vi "PositionInterpolator.vi"() -> ()   [LabVIEW 2013]
panel:
  out "Positions":dbl[](array[numeric])
  in  "timestamp":dbl format="%#_13g"
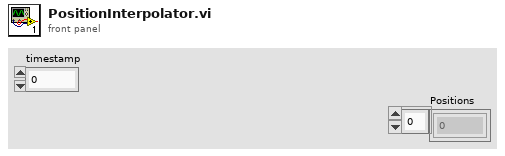
[diagram p1: front panel]
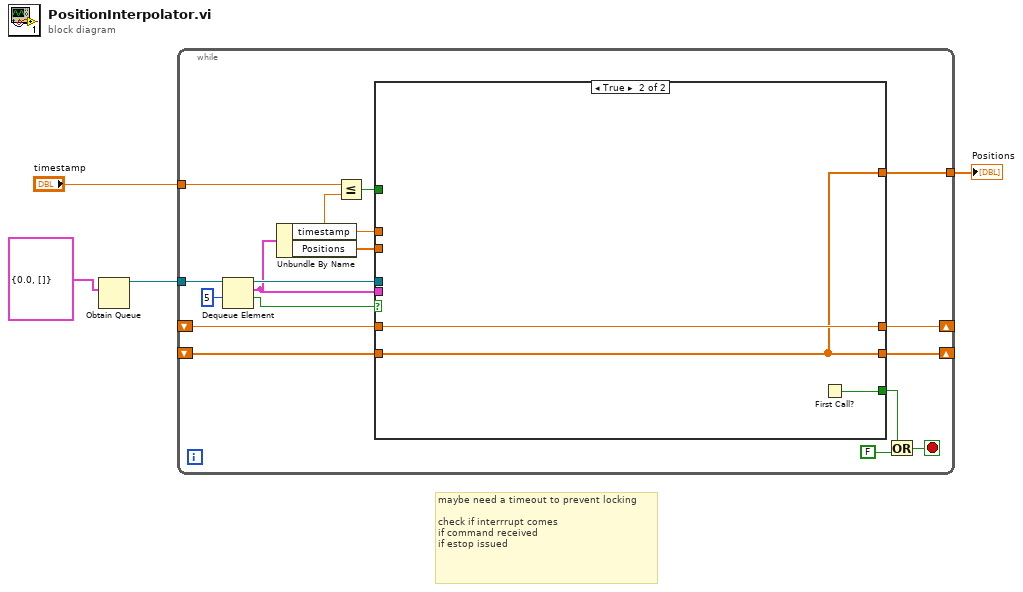
[diagram p0: block diagram]
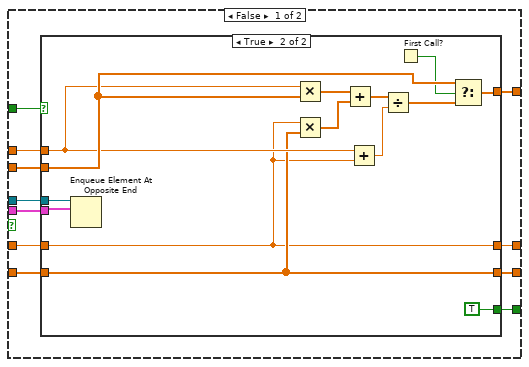
[diagram p2: hidden frame]
diagram:
  # "maybe need a timeout to prevent locking\n\ncheck if interrrupt comes\nif command received\nif estop issued"
  n1 = Obtain Queue(element data type=cluster{"timestamp":dbl, "Positions":dbl[]} {"timestamp"=0.0, "Positions"=[]}) -> (queue out=w3:refnum<queue>)  [unwired: 4 in, 2 out]
  n2 = while {
    tunnel: w3 -> [w21]
    tunnel: "timestamp" -> [w18]
    tunnel: [w14] -> w1
    shift-right: [w12] -> _
    shift-left: _ -> [w9]
    shift-right: [w11] -> _
    shift-left: _ -> [w10]
    stop <- w8 stop-if-true
    n3 = Dequeue Element(queue=w21, timeout in ms (-1)=5) -> (queue out=w20:refnum<queue>, element=w6:cluster{"timestamp":dbl, "Positions":dbl[]}, timed out?=w5:bool)  [unwired: 1 in, 1 out]
    n4 = Unbundle By Name(w6) -> ("timestamp"=w15:dbl, "Positions"=w16:dbl[])
    n5 = Less Or Equal?(x=w18, y=w15) -> (x <= y?=w17:bool)
    n6 = case shown="True" w5 {
      tunnel: w20 -> [w32 _]
      tunnel: w17 -> [w31 _]
      tunnel: w16 -> [w30 _]
      tunnel: w15 -> [w29 _]
      tunnel: [w28 w50] -> w14
      tunnel: [w27 w49] -> w13
      tunnel: [w26 w50] -> w12
      tunnel: [w25 w51] -> w11
      tunnel: w10 -> [w24 w51]
      tunnel: w9 -> [w23 w50]
      tunnel: w6 -> [w22 _]
      frame False {
        n7 = case shown="True" w31 {
          tunnel: w32 -> [_ w36]
          tunnel: w30 -> [w34 w41]
          tunnel: w29 -> [w33 w40]
          tunnel: [_ w43] -> w28
          tunnel: [_ TRUE] -> w27
          tunnel: [w34 w38] -> w26
          tunnel: [w33 w37] -> w25
          tunnel: w24 -> [_ w37]
          tunnel: w23 -> [_ w38]
          tunnel: w22 -> [_ w35]
          frame False {
          }
          frame True {
            n8 = Enqueue Element At Opposite End(queue=w36, element=w35) -> ()  [unwired: 2 in, 3 out]
            n9 = Multiply(x=w40, y=w41) -> (x*y=w48:dbl[])
            n10 = Multiply(x=w37, y=w38) -> (x*y=w47:dbl[])
            n11 = Add(x=w48, y=w47) -> (x+y=w46:dbl[])
            n12 = Add(x=w40, y=w37) -> (x+y=w45:dbl)
            n13 = Divide(x=w46, y=w45) -> (x/y=w44:dbl[])
            n14 = First Call?() -> (First Call?: T/F=w39:bool)
            n15 = Select(t=w41, s=w39, f=w44) -> (s? t:f=w43:dbl[])
          }
        }
      }
      frame True {
        n16 = First Call?() -> (First Call?: T/F=w49:bool)
      }
    }
    n17 = Or(x=w13, y=FALSE) -> (x .or. y?=w8:bool)
  }
  "Positions" <- w1
